vi "2D_check_warning_cw.vi"(0 "val":bool, 1 "validated":string, 3 "ok":bool, 4 "data type":string, 5 "at":bool, 6 "dt":bool, 7 "arr time clock":string, 8 "record interval":string, 9 "ri":bool, 10 "coincidence":string, 11 "co":bool) -> ()   [LabVIEW 2010]
panel:
  # "For 2D operation, you must have:"
  # "Errors"
  # "Current status"
  # "One arrival time clock master\nand one slave."
  # "Only one BSA as master"
  # "The same 'record interval' on\nboth BSA's"
  # "Record the same types of data\non each BSA, which must include \narrival time."
  # "Accept all data (including \nunvalidated data)"
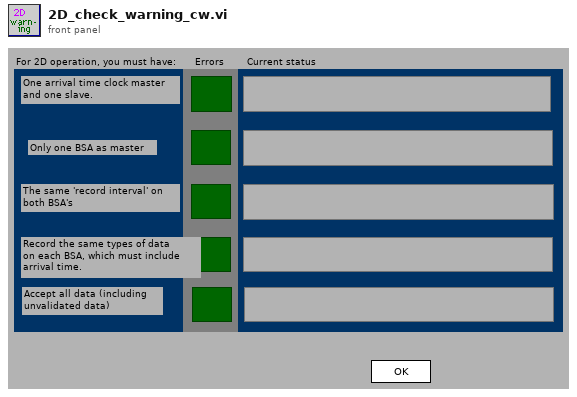
[diagram p1: front panel]
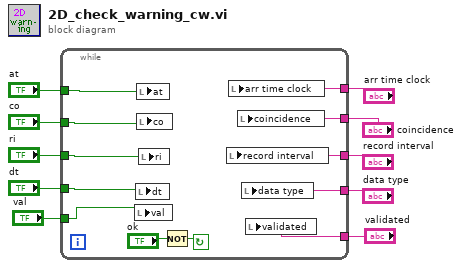
[diagram p0: block diagram]
diagram:
  n1 = while {
    tunnel: "val" -> [w11]
    tunnel: "validated" -> [w12]
    tunnel: "data type" -> [w13]
    tunnel: "record interval" -> [w14]
    tunnel: "coincidence" -> [w15]
    tunnel: "arr time clock" -> [w16]
    tunnel: "dt" -> [w17]
    tunnel: "ri" -> [w18]
    tunnel: "co" -> [w19]
    tunnel: "at" -> [w20]
    stop <- w21 continue-if-true
    n2 = local write "val"(w11) -> ()
    n3 = local write "dt"(w17) -> ()
    n4 = local write "at"(w20) -> ()
    n5 = local write "co"(w19) -> ()
    n6 = local write "ri"(w18) -> ()
    n7 = Not(x="ok") -> (.not. x?=w21:bool)
    n8 = local write "record interval"(w14) -> ()
    n9 = local write "arr time clock"(w16) -> ()
    n10 = local write "coincidence"(w15) -> ()
    n11 = local write "data type"(w13) -> ()
    n12 = local write "validated"(w12) -> ()
  }
